vi "FreqSel.vi"(0 "Ring":u16(ring) items=["0.8 ms", "1.6 ms", "3.2 ms", "6.4 ms", "12.8 ms", "19.2 ms"]) -> (2 "Frequency":u16, 3 "DLY":u16, 4 "SampleTime":sgl)   [LabVIEW 2014]
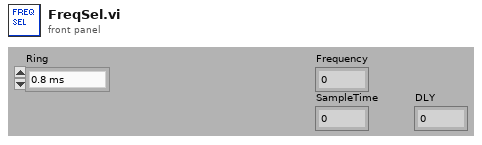
[diagram p1: front panel]
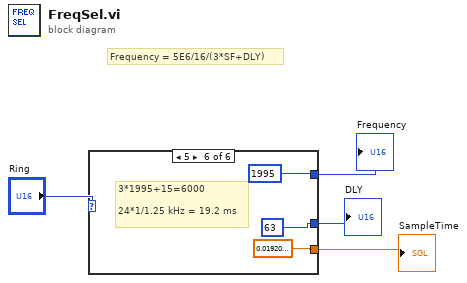
[diagram p0: block diagram]
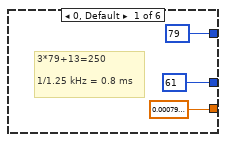
[diagram p2: hidden frame]
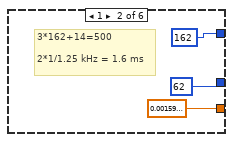
[diagram p3: hidden frame]
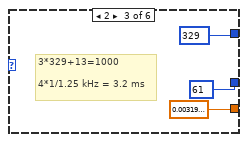
[diagram p4: hidden frame]
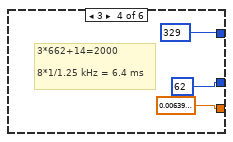
[diagram p5: hidden frame]
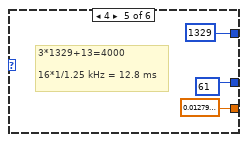
[diagram p6: hidden frame]
diagram:
  # "Frequency = 5E6/16/(3*SF+DLY)"
  n1 = case shown="5" "Ring" {
    tunnel: [u8 79 ("frequenz") u8 162 ("frequenz") u16 329 ("frequenz") u16 329 ("frequenz") u16 1329 ("frequenz") u16 1995 ("frequenz")] -> w2
    tunnel: [u16 61 ("t") u16 62 ("t") u16 61 ("t") u16 62 ("t") u16 61 ("t") u16 63 ("t")] -> w3
    tunnel: [sgl 0.0008 sgl 0.0016 sgl 0.0032 sgl 0.0064 sgl 0.0128 sgl 0.0192] -> w1
    frame 0, Default {
      # "3*79+13=250\n\n1/1.25 kHz = 0.8 ms"
    }
    frame 1 {
      # "3*162+14=500\n\n2*1/1.25 kHz = 1.6 ms"
    }
    frame 2 {
      # "3*329+13=1000\n\n4*1/1.25 kHz = 3.2 ms"
    }
    frame 3 {
      # "3*662+14=2000\n\n8*1/1.25 kHz = 6.4 ms"
    }
    frame 4 {
      # "3*1329+13=4000\n\n16*1/1.25 kHz = 12.8 ms"
    }
    frame 5 {
      # "3*1995+15=6000\n\n24*1/1.25 kHz = 19.2 ms"
    }
  }
  "DLY" <- w3
  "Frequency" <- w2
  "SampleTime" <- w1
